vi "Convolution.vi"() -> ()   [LabVIEW 2022 SP3]
panel:
  out "reversed array":dbl[](array[numeric])
  out "s - size(s)":i32
  out "h - size(s)":i32
  out "Output Vector r":dbl[](array[numeric])
  in  "Input Vector s":dbl[](array[numeric])
  in  "Input Vector h":dbl[](array[numeric])
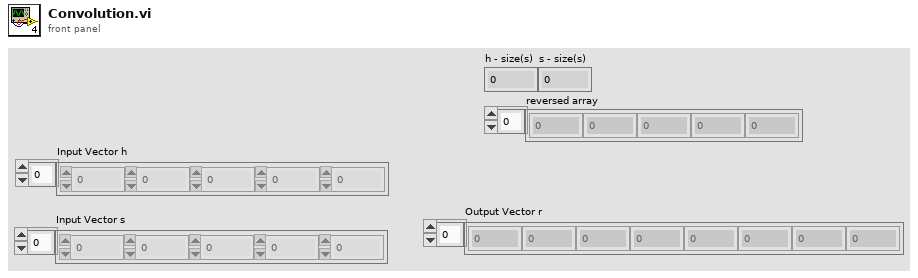
[diagram p1: front panel]
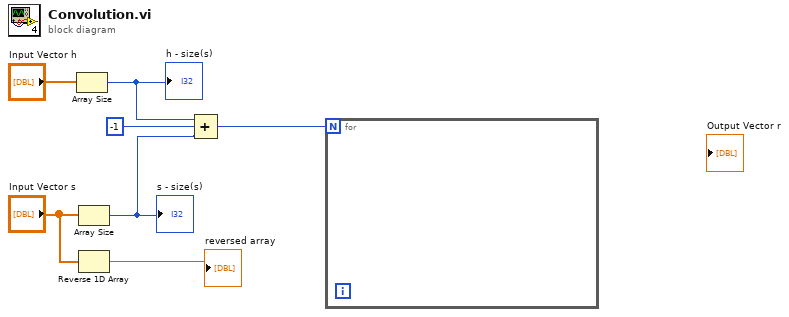
[diagram p0: block diagram]
diagram:
  n1 = Array Size(array="Input Vector h") -> (size(s)=w3:i32)
  "h - size(s)" <- w3
  n2 = Array Size(array="Input Vector s") -> (size(s)=w2:i32)
  "s - size(s)" <- w2
  n3 = Reverse 1D Array(array="Input Vector s") -> (reversed array=→"reversed array":dbl[])
  n4 = Compound Arithmetic op=ADD(w3, -1, w2) -> (w5:i32)
  n5 = for {
    N: w5 -> [_]
  }
